vi "Save Best Fit Parameters.vi"(8 "Current File Num":u16, 9 "Best Fit Parameters":dbl[](array[numeric]), 10 "Fitting Results Save Path":string[](array[string]), 11 "Fitting Type":u16(ring)) -> ()   [LabVIEW 2015]
uses:
  <vilib>/Utility/file.llb/Read From Spreadsheet File (DBL).vi
  <vilib>/Utility/file.llb/Write To Spreadsheet File (DBL).vi
panel:
  out "Best Fit Parameters 2":dbl[](array[numeric])
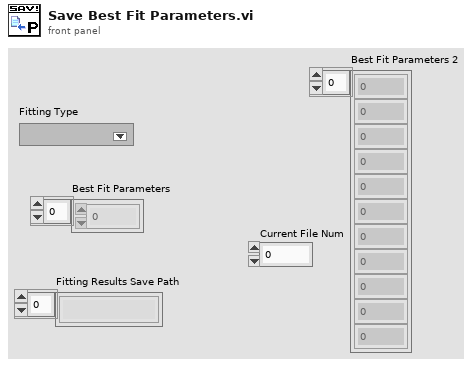
[diagram p1: front panel]
types:
  T1 = enum16{"open", "replace", "create", "open or create", "replace or create", "replace or create with confirmation"}
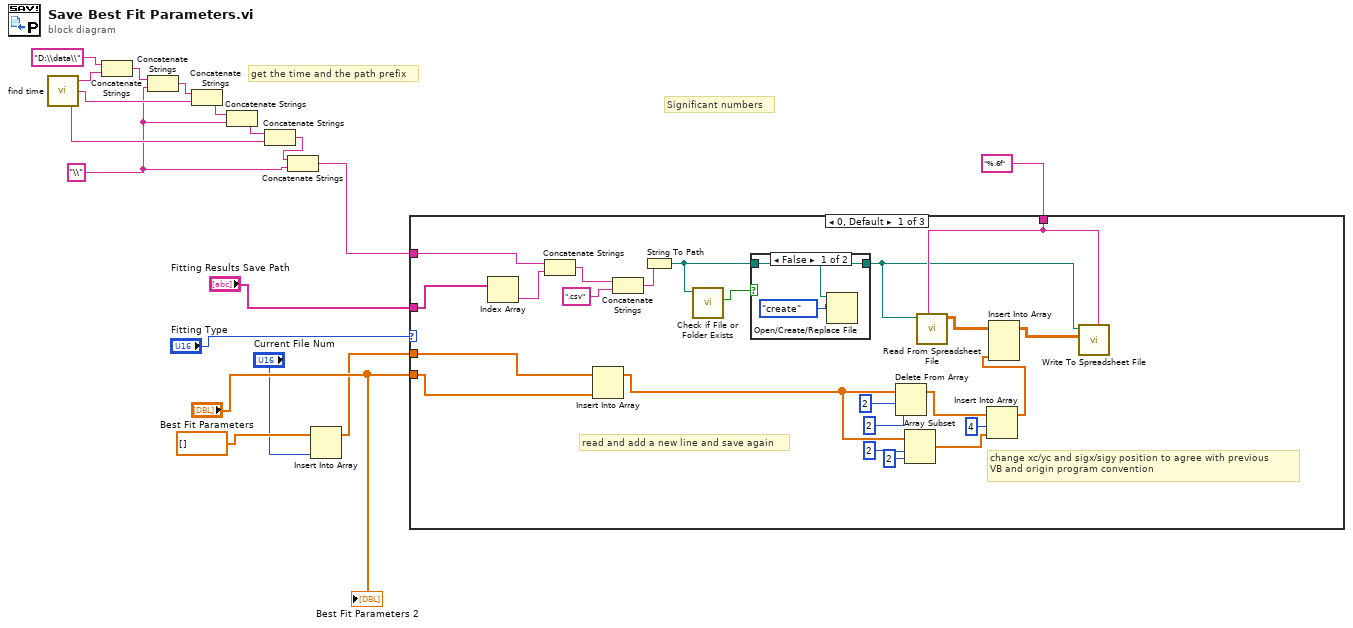
[diagram p0: block diagram]
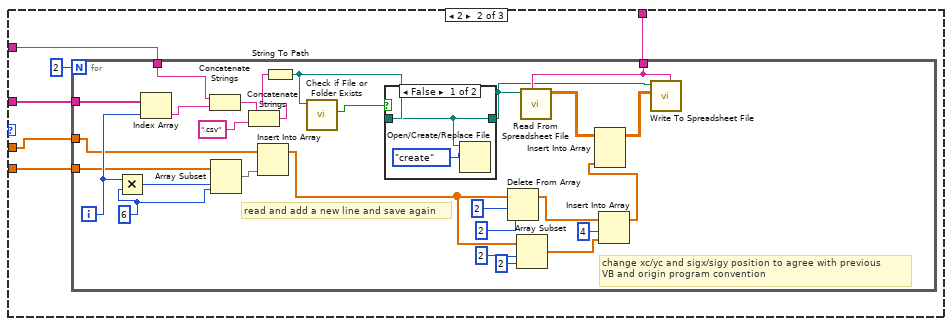
[diagram p3: hidden frame]
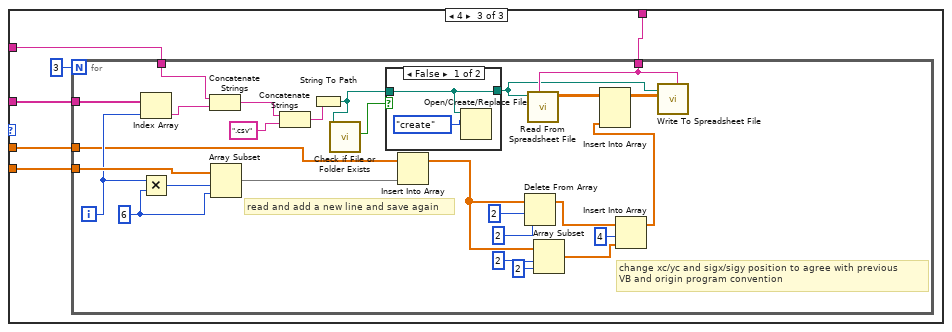
[diagram p5: hidden frame]
diagram:
  w2 = "\\" ("字符串")
  # "get the time and the path prefix"
  # "Significant numbers"
  n1 = call "find time.vi"() -> ("day"=w4:string, "month"=w7:string, "year"=w10:string)  [unwired: 3 in]
  n2 = Concatenate Strings("D:\\data\\", w10) -> (w9:string)
  n3 = Concatenate Strings(w9, w2) -> (w8:string)
  n4 = Concatenate Strings(w8, w7) -> (w6:string)
  n5 = Concatenate Strings(w6, w2) -> (w5:string)
  n6 = Concatenate Strings(w5, w4) -> (w3:string)
  n7 = Concatenate Strings(w3, w2) -> (w1:string)
  n8 = Insert Into Array(array=dbl[] [], new element="Current File Num") -> (w13:dbl[])  [unwired: 1 in]
  n9 = case shown="0, Default" "Fitting Type" {
    tunnel: "Best Fit Parameters" -> [w36 w49 w85]
    tunnel: "Fitting Results Save Path" -> [w39 w48 w84]
    tunnel: w13 -> [w37 w47 w83]
    tunnel: "%.6f" ("format (%.3f)") -> [w35 w46 w82]
    tunnel: w1 -> [w34 w45 w81]
    frame 0, Default {
      # "change xc/yc and sigx/sigy position to agree with previous\nVB and origin program convention"
      # "read and add a new line and save again"
      n10 = Index Array(array=w39) -> (element=w38:string)  [unwired: 1 in]
      n11 = Concatenate Strings(w34, w38) -> (w32:string)
      n12 = Insert Into Array(array=w37, new element=w36) -> (w25:dbl[])  [unwired: 1 in]
      n13 = Concatenate Strings(w32, ".csv" ("字符串")) -> (w31:string)
      n14 = String To Path(string=w31) -> (path=w30:path)
      n15 = call <vilib>:"Check if File or Folder Exists.vi"("path"=w30) -> ("file or folder exists?"=w28:bool)  [unwired: 8 in, 2 out]
      n16 = case shown="False" w28 {
        tunnel: w30 -> [w42 w44]
        tunnel: [w42 w44] -> w29
        frame False {
          n17 = Open/Create/Replace File(file path (use dialog)=w42, operation (0:open)=T1."create" ("操作(0:open)")) -> ()  [unwired: 4 in, 3 out]
        }
        frame True {
        }
      }
      n18 = Delete From Array(array=w25, length=2, index=2) -> (array with subset deleted=w22:dbl[])  [unwired: 1 out]
      n19 = Array Subset(array=w25, index=2, length=2) -> (w20:dbl[])
      n20 = call-poly <vilib>:"Read From Spreadsheet File.vi"("format (%.3f)"=w35, "file path (dialog if empty)"=w29) -> ("all rows"=w41:dbl[][])  [unwired: 5 in, 4 out]
      n21 = Insert Into Array(array=w22, index=4, new element=w20) -> (w19:dbl[])
      n22 = Insert Into Array(array=w41, new element=w19) -> (w40:dbl[][])  [unwired: 2 in]
      n23 = call-poly <vilib>:"Write To Spreadsheet File.vi"("format (%.3f)"=w35, "2D data"=w40, "file path (dialog if empty)"=w29) -> ()  [unwired: 5 in, 1 out]
    }
    frame 2 {
      n24 = for {
        N: 2 -> [_]
        tunnel: w49 -> [w69]
        tunnel: w48 -> [w75]
        tunnel: w47 -> [w70]
        tunnel: w46 -> [w67]
        tunnel: w45 -> [w66]
        i -> [w74]
        w76 = 6 ("x")
        # "change xc/yc and sigx/sigy position to agree with previous\nVB and origin program convention"
        # "read and add a new line and save again"
        n25 = Multiply(x=w74, y=w76) -> (x*y=w77:i32)
        n26 = Index Array(array=w75, index=w74) -> (element=w73:string)
        n27 = Concatenate Strings(w66, w73) -> (w65:string)
        n28 = Array Subset(array=w69, index=w77, length=w76) -> (w68:dbl[])
        n29 = Concatenate Strings(w65, ".csv" ("字符串")) -> (w63:string)
        n30 = Insert Into Array(array=w70, new element=w68) -> (w52:dbl[])  [unwired: 1 in]
        n31 = String To Path(string=w63) -> (path=w62:path)
        n32 = call <vilib>:"Check if File or Folder Exists.vi"("path"=w62) -> ("file or folder exists?"=w60:bool)  [unwired: 8 in, 2 out]
        n33 = case shown="False" w60 {
          tunnel: w62 -> [w78 w80]
          tunnel: [w78 w80] -> w61
          frame False {
            n34 = Open/Create/Replace File(file path (use dialog)=w78, operation (0:open)=T1."create" ("操作(0:open)")) -> ()  [unwired: 4 in, 3 out]
          }
          frame True {
          }
        }
        n35 = Delete From Array(array=w52, length=2, index=2) -> (array with subset deleted=w55:dbl[])  [unwired: 1 out]
        n36 = Array Subset(array=w52, index=2, length=2) -> (w53:dbl[])
        n37 = call-poly <vilib>:"Read From Spreadsheet File.vi"("format (%.3f)"=w67, "file path (dialog if empty)"=w61) -> ("all rows"=w72:dbl[][])  [unwired: 5 in, 4 out]
        n38 = Insert Into Array(array=w55, index=4, new element=w53) -> (w51:dbl[])
        n39 = Insert Into Array(array=w72, new element=w51) -> (w71:dbl[][])  [unwired: 2 in]
        n40 = call-poly <vilib>:"Write To Spreadsheet File.vi"("format (%.3f)"=w67, "2D data"=w71, "file path (dialog if empty)"=w61) -> ()  [unwired: 5 in, 1 out]
      }
    }
    frame 4 {
      n41 = for {
        N: 3 -> [_]
        tunnel: w85 -> [w111]
        tunnel: w84 -> [w110]
        tunnel: w83 -> [w104]
        tunnel: w82 -> [w103]
        tunnel: w81 -> [w102]
        i -> [w109]
        w112 = 6 ("x")
        # "change xc/yc and sigx/sigy position to agree with previous\nVB and origin program convention"
        # "read and add a new line and save again"
        n42 = Index Array(array=w110, index=w109) -> (element=w108:string)
        n43 = Multiply(x=w109, y=w112) -> (x*y=w113:i32)
        n44 = Concatenate Strings(w102, w108) -> (w100:string)
        n45 = Array Subset(array=w111, index=w113, length=w112) -> (w105:dbl[])
        n46 = Concatenate Strings(w100, ".csv" ("字符串")) -> (w99:string)
        n47 = String To Path(string=w99) -> (path=w97:path)
        n48 = call <vilib>:"Check if File or Folder Exists.vi"("path"=w97) -> ("file or folder exists?"=w98:bool)  [unwired: 8 in, 2 out]
        n49 = case shown="False" w98 {
          tunnel: [w114 w116] -> w96
          tunnel: w97 -> [w114 w116]
          frame False {
            n50 = Open/Create/Replace File(file path (use dialog)=w114, operation (0:open)=T1."create" ("操作(0:open)")) -> ()  [unwired: 4 in, 3 out]
          }
          frame True {
          }
        }
        n51 = Insert Into Array(array=w104, new element=w105) -> (w88:dbl[])  [unwired: 1 in]
        n52 = Delete From Array(array=w88, length=2, index=2) -> (array with subset deleted=w91:dbl[])  [unwired: 1 out]
        n53 = call-poly <vilib>:"Read From Spreadsheet File.vi"("format (%.3f)"=w103, "file path (dialog if empty)"=w96) -> ("all rows"=w107:dbl[][])  [unwired: 5 in, 4 out]
        n54 = Array Subset(array=w88, index=2, length=2) -> (w89:dbl[])
        n55 = Insert Into Array(array=w91, index=4, new element=w89) -> (w87:dbl[])
        n56 = Insert Into Array(array=w107, new element=w87) -> (w106:dbl[][])  [unwired: 2 in]
        n57 = call-poly <vilib>:"Write To Spreadsheet File.vi"("format (%.3f)"=w103, "2D data"=w106, "file path (dialog if empty)"=w96) -> ()  [unwired: 5 in, 1 out]
      }
    }
  }
  "Best Fit Parameters 2" <- "Best Fit Parameters"
